vi "Check Valid.vi"(11 "AbstractLogMessage.lvclass":refnum<class "AbstractLogMessage.lvclass">) -> (3 "Valid?":bool)   [LabVIEW 2020]
uses:
  AbstractLogMessage.lvclass
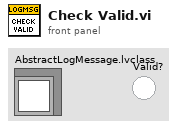
[diagram p1: front panel]
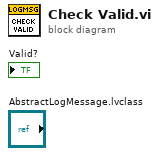
[diagram p0: block diagram]
diagram:
